vi "Save Banking Records.vi"(8 "error in (no error)":errorcluster, 9 "Importing Transactions":refnum<class "Statement.lvclass">, 10 "Overlapping Records":refnum<class "Statement.lvclass">, 11 "Database in":refnum<class "Database.lvclass">) -> (0 "error out":errorcluster, 3 "Database out":refnum<class "Database.lvclass">)   [LabVIEW 2018, in "Database.lvclass"]
uses:
  Database.lvclass
  Statement/Statement.lvclass
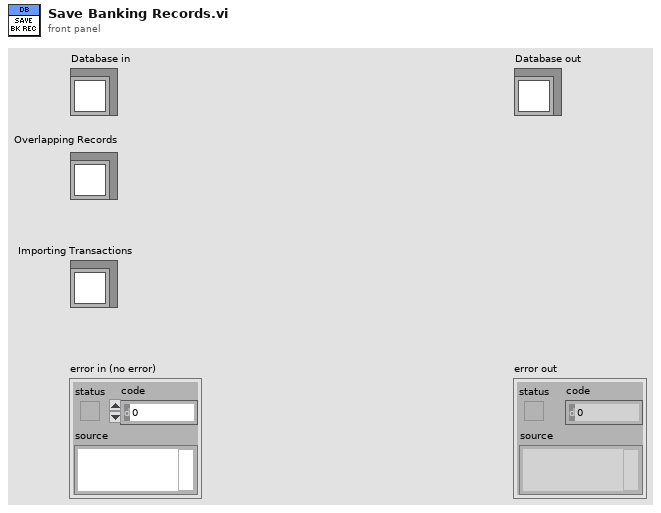
[diagram p1: front panel]
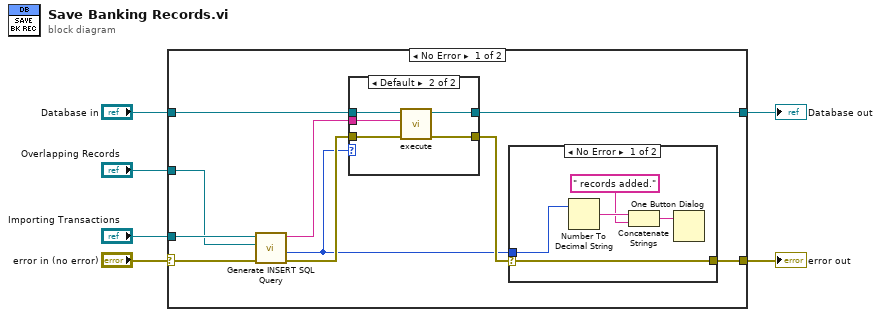
[diagram p0: block diagram]
diagram:
  n1 = case shown="No Error" "error in (no error)" {
    selector: "error in (no error)" -> [w13 w31]
    tunnel: [w9 w31] -> w5
    tunnel: [w15 w30] -> w3
    tunnel: "Database in" -> [w16 w30]
    tunnel: "Importing Transactions" -> [w14 _]
    tunnel: "Overlapping Records" -> [w12 _]
    frame No Error {
      n2 = call-dynamic "Generate INSERT SQL Query.vi"("error in (no error)"=w13, "Overlappping Records"=w12, "Importing Transactions"=w14) -> ("error out"=w11:errorcluster, "Num records"=w8:i32, "INSERT Query"=w7:string)  [unwired: 6 in]
      n3 = case shown="Default" w8 {
        tunnel: w16 -> [w24 w29]
        tunnel: [w24 w28] -> w15
        tunnel: w11 -> [w23 w27]
        tunnel: [w23 w25] -> w10
        tunnel: w7 -> [_ w26]
        frame 0 {
        }
        frame Default {
          n4 = call "execute.vi"("error in (no error)"=w27, "SQL query"=w26, "Database in"=w29) -> ("error out"=w25:errorcluster, "Database out"=w28:refnum<class "Database.lvclass">)  [unwired: 7 in]
        }
      }
      n5 = case shown="No Error" w10 {
        selector: w10 -> [w18 w22]
        tunnel: [w18 w22] -> w9
        tunnel: w8 -> [w17 _]
        frame No Error {
          n6 = Number To Decimal String(number=w17) -> (decimal integer string=w20:string)  [unwired: 1 in]
          n7 = Concatenate Strings(w20, " records added.") -> (w21:string)
          n8 = One Button Dialog(message=w21) -> ()  [unwired: 1 in, 1 out]
        }
        frame Error {
        }
      }
    }
    frame Error {
    }
  }
  "error out" <- w5
  "Database out" <- w3
